vi "PWM set.vi"(4 "Motor.brake":bool, 6 "Reset":bool, 7 "pwm cnfg":T1, 8 "Error In":errorcluster, 9 "motor select":T2, 10 "PWM":dbl, 11 "FPGA VI Reference In":refnum<k20>) -> (0 "error out":errorcluster)   [LabVIEW 2019, in "my FPGA lib.lvlib" / "motor.lvlib"]
uses:
  motor.lvlib
  motor enum.ctl
  <vilib>/Utility/error.llb/Error Cluster From Error Code.vi
  <vilib>/rvi/errors/niLvFpgaAdjustHostInterfaceError.vi
  <vilib>/rvi/interface/nirviReadWriteControl/nirviReadWriteControl.xnode
  NiFpgaLv.dll
  <vilib>/rvi/interface/Simulation/niFpgaSimulationCallBeginRW.vi
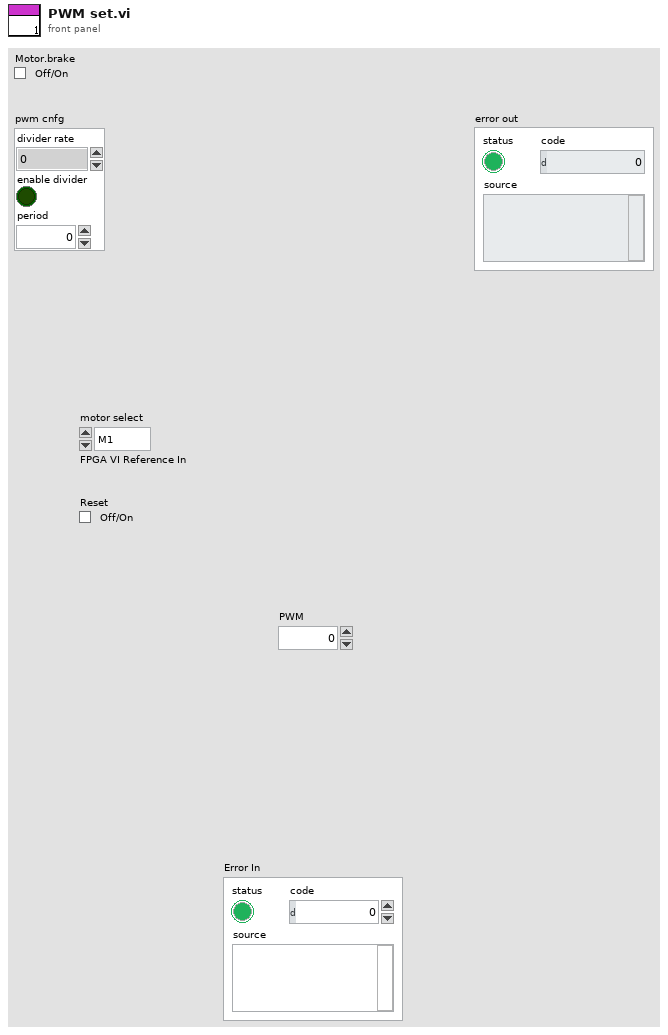
[diagram p1: front panel]
types:
  T1 = cluster{"divider rate":i32, "enable divider":bool, "period":i32}
  T2 = typedef "my FPGA lib.lvlib/motor.lvlib/motor enum.ctl" = enum16{"M1", "M2", "M3", "M4"}
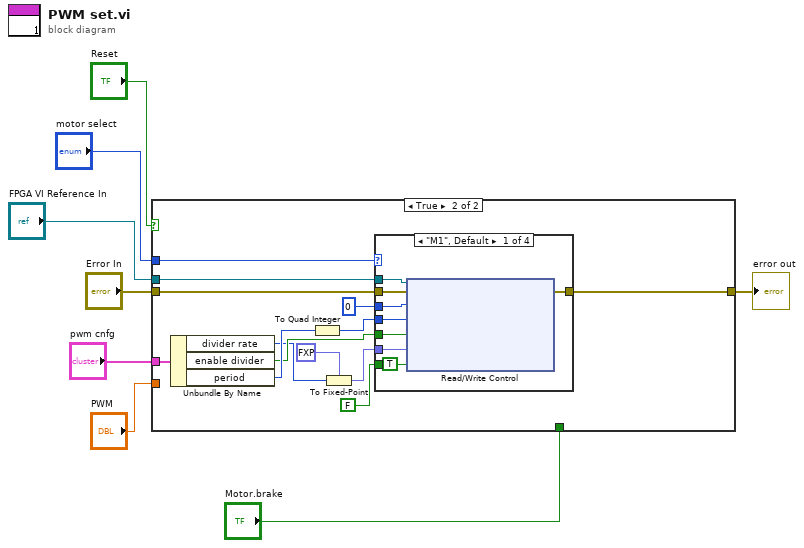
[diagram p0: block diagram]
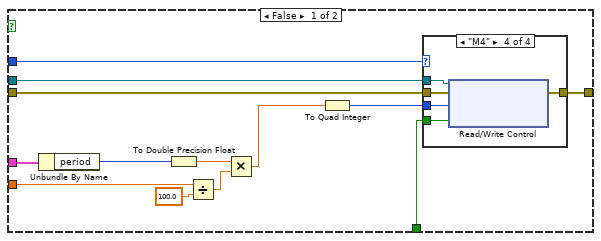
[diagram p2: hidden frame]
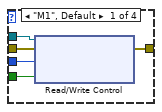
[diagram p3: hidden frame]
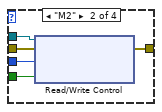
[diagram p4: hidden frame]
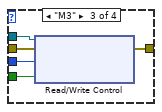
[diagram p5: hidden frame]
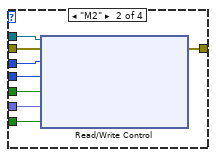
[diagram p6: hidden frame]
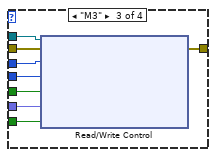
[diagram p7: hidden frame]
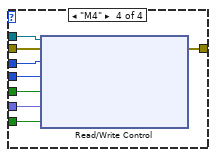
[diagram p8: hidden frame]
diagram:
  n1 = case shown="True" "Reset" {
    tunnel: "motor select" -> [w14 w54]
    tunnel: "Error In" -> [w12 w53]
    tunnel: "FPGA VI Reference In" -> [w13 w52]
    tunnel: "pwm cnfg" -> [w19 w50]
    tunnel: [w10 w42] -> w3
    tunnel: "PWM" -> [w21 _]
    tunnel: "Motor.brake" -> [w9 _]
    frame False {
      n2 = Unbundle By Name(w19) -> ("period"=w18:i32)
      n3 = To Double Precision Float(number=w18) -> (double precision float=w17:dbl)
      n4 = Divide(x=w21, y=100.0) -> (x/y=w16:dbl)
      n5 = Multiply(x=w17, y=w16) -> (x*y=w15:dbl)
      n6 = To Quad Integer(1:w15) -> (0:w11:i64)
      n7 = case shown="\"M4\"" w14 {
        tunnel: w13 -> [w26 w31 w36 w41]
        tunnel: w12 -> [w25 w30 w35 w40]
        tunnel: w9 -> [w24 w29 w34 w39]
        tunnel: w11 -> [w23 w28 w33 w38]
        tunnel: [w22 w27 w32 w37] -> w10
        frame "M1", Default {
          n8 = xnode "Read/Write Control"("FPGA VI Reference In"=w26, "error in"=w25, "Motor1.speed"=w23, "Motor1.brake"=w24) -> ("error out"=w22:errorcluster)  [unwired: 1 out]
        }
        frame "M2" {
          n9 = xnode "Read/Write Control"("FPGA VI Reference In"=w31, "error in"=w30, "Motor2.speed"=w28, "Motor2.brake"=w29) -> ("error out"=w27:errorcluster)  [unwired: 1 out]
        }
        frame "M3" {
          n10 = xnode "Read/Write Control"("FPGA VI Reference In"=w36, "error in"=w35, "Motor3.speed"=w33, "Motor3.brake"=w34) -> ("error out"=w32:errorcluster)  [unwired: 1 out]
        }
        frame "M4" {
          n11 = xnode "Read/Write Control"("FPGA VI Reference In"=w41, "error in"=w40, "Motor4.speed"=w38, "Motor4.brake"=w39) -> ("error out"=w37:errorcluster)  [unwired: 1 out]
        }
      }
    }
    frame True {
      n12 = Unbundle By Name(w50) -> ("divider rate"=w45:i32, "enable divider"=w46:bool, "period"=w49:i32)
      n13 = To Quad Integer(1:w49) -> (0:w48:i64)
      n14 = To Fixed-Point(fixed-point type=fxp<+,4,4> 0.0 ("Motor1.divider"), number=w45) -> (fixed-point=w43:fxp<+,4,4>)
      n15 = case shown="\"M1\", Default" w54 {
        tunnel: w53 -> [w62 w70 w78 w86]
        tunnel: w52 -> [w61 w69 w77 w85]
        tunnel: FALSE ("Motor1.brake") -> [_ w68 w76 w84]
        tunnel: w48 -> [w60 w67 w75 w83]
        tunnel: i64 0 ("Motor1.speed") -> [w59 w66 w74 w82]
        tunnel: w46 -> [w58 w65 w73 w81]
        tunnel: w43 -> [w57 w64 w72 w80]
        tunnel: [w56 w63 w71 w79] -> w42
        frame "M1", Default {
          n16 = xnode "Read/Write Control"("FPGA VI Reference In"=w61, "error in"=w62, "Motor1.speed"=w59, "Motor1.periode"=w60, "Motor1.enable_divider"=w58, "Motor1.divider"=w57, "Motor1.brake"=TRUE) -> ("error out"=w56:errorcluster)  [unwired: 1 out]
        }
        frame "M2" {
          n17 = xnode "Read/Write Control"("FPGA VI Reference In"=w69, "error in"=w70, "Motor2.speed"=w66, "Motor2.periode"=w67, "Motor2.enable_divider"=w65, "Motor2.divider"=w64, "Motor2.brake"=w68) -> ("error out"=w63:errorcluster)  [unwired: 1 out]
        }
        frame "M3" {
          n18 = xnode "Read/Write Control"("FPGA VI Reference In"=w77, "error in"=w78, "Motor3.speed"=w74, "Motor3.periode"=w75, "Motor3.enable_divider"=w73, "Motor3.divider"=w72, "Motor3.brake"=w76) -> ("error out"=w71:errorcluster)  [unwired: 1 out]
        }
        frame "M4" {
          n19 = xnode "Read/Write Control"("FPGA VI Reference In"=w85, "error in"=w86, "Motor4.speed"=w82, "Motor4.periode"=w83, "Motor4.enable_divider"=w81, "Motor4.divider"=w80, "Motor4.brake"=w84) -> ("error out"=w79:errorcluster)  [unwired: 1 out]
        }
      }
    }
  }
  "error out" <- w3
